vi "AB_820_850_CheckForValidExtension.vi"(9 "buildType":T1, 11 "Filename in":string) -> (1 "ChangedExtension?":bool, 3 "Filename out":string)   [LabVIEW 2020]
uses:
  <vilib>/AppBuilder/AB_BuildType.ctl
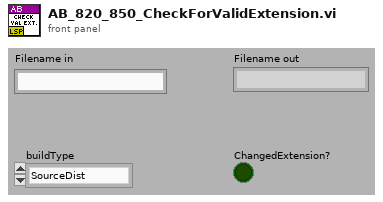
[diagram p1: front panel]
types:
  T1 = typedef "AB_BuildType.ctl" = enum16{"SourceDist", "EXE", "DLL", "RTExe"}
  T2 = enum32{"invalid OS target", "Mac OS", "Windows 3.1", "Windows 95/NT", "Solaris 1", "Solaris 2", "HP-UX", "PowerMAX", "Linux", "Irix", "Rhapsody", "BeOS", "AIX", "OSF1", "VxWorks", "PharLap", "Carbon", "RTX", "Windows x64", "Linux x64", "Mac OS X x64"}
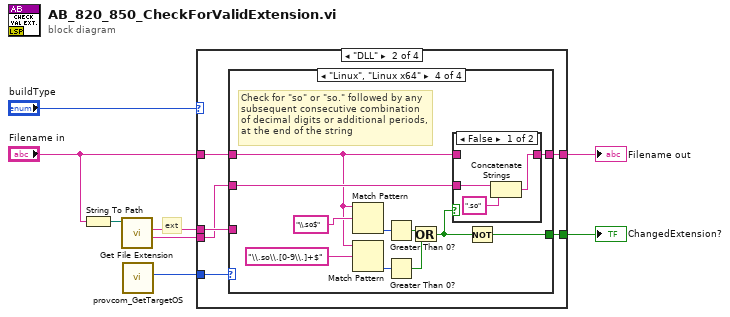
[diagram p0: block diagram]
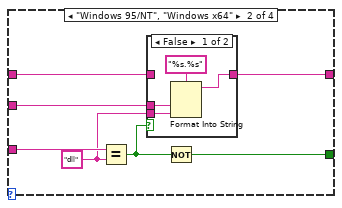
[diagram p4: hidden frame]
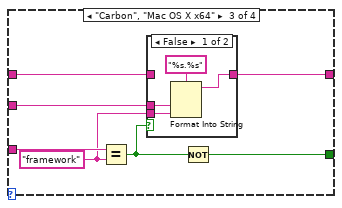
[diagram p6: hidden frame]
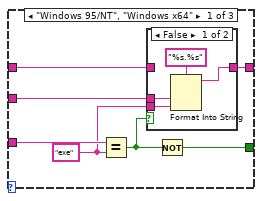
[diagram p10: hidden frame]
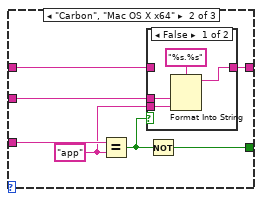
[diagram p12: hidden frame]
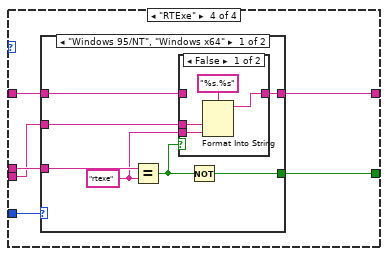
[diagram p14: hidden frame]
diagram:
  # "ext"
  n1 = String To Path(string="Filename in") -> (path=w6:path)
  n2 = call <vilib>:"Get File Extension.vi"("file"=w6) -> ("filename without extension"=w8:string, "lowercase file extension"=w7:string)  [unwired: 6 in, 3 out]
  n3 = call <resource>:"provcom_GetTargetOS.vi"() -> ("App.TargetOS"=w1:T2)  [unwired: 11 in]
  n4 = case shown="\"DLL\"" "buildType" {
    tunnel: w1 -> [_ w15 w61 w92]
    tunnel: "Filename in" -> [w9 w14 w60 w91]
    tunnel: [_ w13 w59 w90] -> w2
    tunnel: w7 -> [_ w12 w58 w89]
    tunnel: w8 -> [_ w11 w57 w88]
    tunnel: [w9 w10 w56 w87] -> w3
    frame Default {
      # "Since this VI is usually called by App class build types (EXE and DLL), Source Dist code should not call this VI. But adding explicit case to pass input through just in case."
    }
    frame "DLL" {
      n5 = case shown="\"Linux\", \"Linux x64\"" w15 {
        tunnel: w14 -> [w16 w22 w34 w42]
        tunnel: [_ w17 w29 w41] -> w13
        tunnel: w11 -> [_ w20 w32 w45]
        tunnel: [w16 w21 w33 w44] -> w10
        tunnel: w12 -> [_ w23 w35 _]
        frame Default {
          # "For unknown OS's, just pass the filename through."
        }
        frame "Windows 95/NT", "Windows x64" {
          w19 = "dll"
          n6 = Equal?(x=w23, y=w19) -> (x = y?=w18:bool)
          n7 = case shown="False" w18 {
            tunnel: w20 -> [w26 _]
            tunnel: w19 -> [w25 _]
            tunnel: w22 -> [_ w28]
            tunnel: [w24 w28] -> w21
            frame False {
              n8 = Format Into String(format string="%s.%s", w26, w25) -> (resulting string=w24:string)  [unwired: 2 in, 1 out]
            }
            frame True {
            }
          }
          n9 = Not(x=w18) -> (.not. x?=w17:bool)
        }
        frame "Carbon", "Mac OS X x64" {
          w31 = "framework"
          n10 = Equal?(x=w35, y=w31) -> (x = y?=w30:bool)
          n11 = case shown="False" w30 {
            tunnel: w32 -> [w38 _]
            tunnel: w31 -> [w37 _]
            tunnel: w34 -> [_ w40]
            tunnel: [w36 w40] -> w33
            frame False {
              n12 = Format Into String(format string="%s.%s", w38, w37) -> (resulting string=w36:string)  [unwired: 2 in, 1 out]
            }
            frame True {
            }
          }
          n13 = Not(x=w30) -> (.not. x?=w29:bool)
        }
        frame "Linux", "Linux x64" {
          # "Check for \"so\" or \"so.\" followed by any subsequent consecutive combination of decimal digits or additional periods, at the end of the string"
          n14 = Match Pattern(string=w42, regular expression="\\.so$") -> (offset past match=w49:i32)  [unwired: 1 in, 3 out]
          n15 = Match Pattern(string=w42, regular expression="\\.so\\.[0-9\\.]+$") -> (offset past match=w48:i32)  [unwired: 1 in, 3 out]
          n16 = Greater Than 0?(x=w49) -> (x > 0?=w47:bool)
          n17 = Greater Than 0?(x=w48) -> (x > 0?=w46:bool)
          n18 = Or(x=w47, y=w46) -> (x .or. y?=w43:bool)
          n19 = case shown="False" w43 {
            tunnel: w45 -> [w54 _]
            tunnel: w42 -> [_ w55]
            tunnel: [w53 w55] -> w44
            frame False {
              n20 = Concatenate Strings(w54, ".so" ("string")) -> (w53:string)
            }
            frame True {
            }
          }
          n21 = Not(x=w43) -> (.not. x?=w41:bool)
        }
      }
    }
    frame "EXE" {
      n22 = case shown="\"Linux\", \"Linux x64\", Default" w61 {
        tunnel: w60 -> [w64 w79 w86]
        tunnel: [w62 w74 _] -> w59
        tunnel: w58 -> [w68 w80 _]
        tunnel: w57 -> [w67 w77 _]
        tunnel: [w63 w78 w86] -> w56
        frame "Windows 95/NT", "Windows x64" {
          w66 = "exe"
          n23 = Equal?(x=w68, y=w66) -> (x = y?=w65:bool)
          n24 = case shown="False" w65 {
            tunnel: w67 -> [w71 _]
            tunnel: w66 -> [w70 _]
            tunnel: w64 -> [_ w73]
            tunnel: [w69 w73] -> w63
            frame False {
              n25 = Format Into String(format string="%s.%s", w71, w70) -> (resulting string=w69:string)  [unwired: 2 in, 1 out]
            }
            frame True {
            }
          }
          n26 = Not(x=w65) -> (.not. x?=w62:bool)
        }
        frame "Carbon", "Mac OS X x64" {
          w76 = "app"
          n27 = Equal?(x=w80, y=w76) -> (x = y?=w75:bool)
          n28 = case shown="False" w75 {
            tunnel: w77 -> [w83 _]
            tunnel: w76 -> [w82 _]
            tunnel: w79 -> [_ w85]
            tunnel: [w81 w85] -> w78
            frame False {
              n29 = Format Into String(format string="%s.%s", w83, w82) -> (resulting string=w81:string)  [unwired: 2 in, 1 out]
            }
            frame True {
            }
          }
          n30 = Not(x=w75) -> (.not. x?=w74:bool)
        }
        frame "Linux", "Linux x64", Default {
          # "For Linux and unknown OS's, just pass the filename through."
        }
      }
    }
    frame "RTExe" {
      n31 = case shown="\"Windows 95/NT\", \"Windows x64\"" w92 {
        tunnel: w91 -> [w95 w105]
        tunnel: [w93 _] -> w90
        tunnel: w89 -> [w99 _]
        tunnel: w88 -> [w98 _]
        tunnel: [w94 w105] -> w87
        frame "Windows 95/NT", "Windows x64" {
          w97 = "rtexe"
          n32 = Equal?(x=w99, y=w97) -> (x = y?=w96:bool)
          n33 = case shown="False" w96 {
            tunnel: w98 -> [w102 _]
            tunnel: w97 -> [w101 _]
            tunnel: w95 -> [_ w104]
            tunnel: [w100 w104] -> w94
            frame False {
              n34 = Format Into String(format string="%s.%s", w102, w101) -> (resulting string=w100:string)  [unwired: 2 in, 1 out]
            }
            frame True {
            }
          }
          n35 = Not(x=w96) -> (.not. x?=w93:bool)
        }
        frame Default {
          # "For unknown OS's, just pass the filename through."
        }
      }
    }
  }
  "ChangedExtension?" <- w2
  "Filename out" <- w3
